vi "Random Number Generation.vi"() -> (8 "number (0 to 1) 2":dbl, 9 "number (0 to 1)":dbl)   [LabVIEW 2018]
doc: "Vi for creating random number in range of 0 --> 1"
panel:
  in  "stop 2":bool
  in  "stop":bool
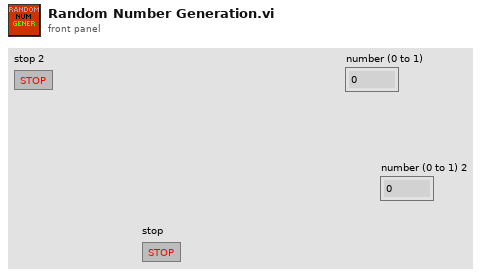
[diagram p1: front panel]
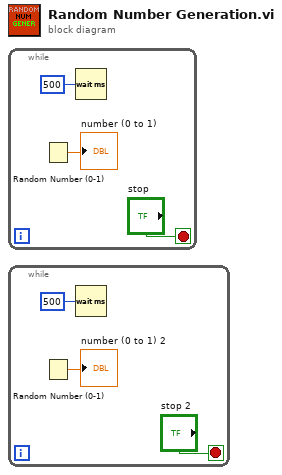
[diagram p0: block diagram]
diagram:
  n1 = while {
    stop <- "stop" stop-if-true
    n2 = Random Number (0-1)() -> (number: 0 to 1=→"number (0 to 1)":dbl)
    n3 = Wait (ms)(milliseconds to wait=u32 500) -> ()  [unwired: 1 out]
  }
  n4 = while {
    stop <- "stop 2" stop-if-true
    n5 = Random Number (0-1)() -> (number: 0 to 1=→"number (0 to 1) 2":dbl)
    n6 = Wait (ms)(milliseconds to wait=u32 500) -> ()  [unwired: 1 out]
  }
